vi "json To Pretty String.vi"   [LabVIEW 2016, in "JSON Document.lvclass"]
uses:
  JSON Document.lvclass
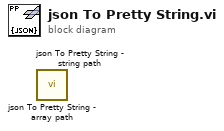
[diagram p0: block diagram]
diagram:
  n1 = call "json To Pretty String - array path.vi"() -> ()  [unwired: 9 in, 3 out]
  n2 = call "json To Pretty String - string path.vi"() -> ()  [unwired: 9 in, 3 out]
